vi "MaqEst.vi"() -> ()   [LabVIEW 2020]
uses:
  idle.ctl
panel:
  out "Dispensar":bool
  out "Enum 2":T1
  out "Dar Cambio":bool
  in  "Selected":bool
  in  "Coin Inserted":bool
  in  "Enough Coins":bool
  in  "Cancel":bool
  in  "Reject coins":bool
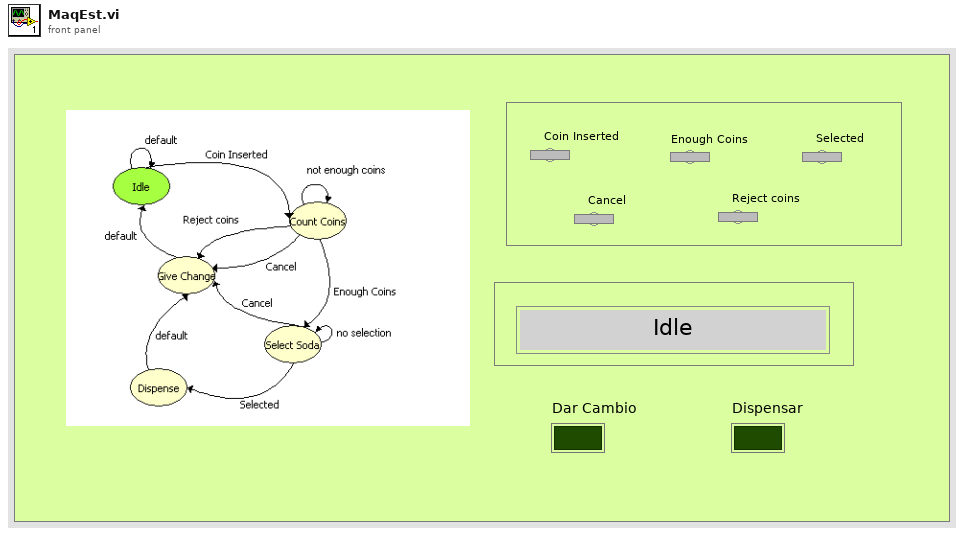
[diagram p1: front panel]
types:
  T1 = typedef "idle.ctl" = enum16{"Idle", "Count Coins", "Give Change", "Select Soda", "Dispense"}
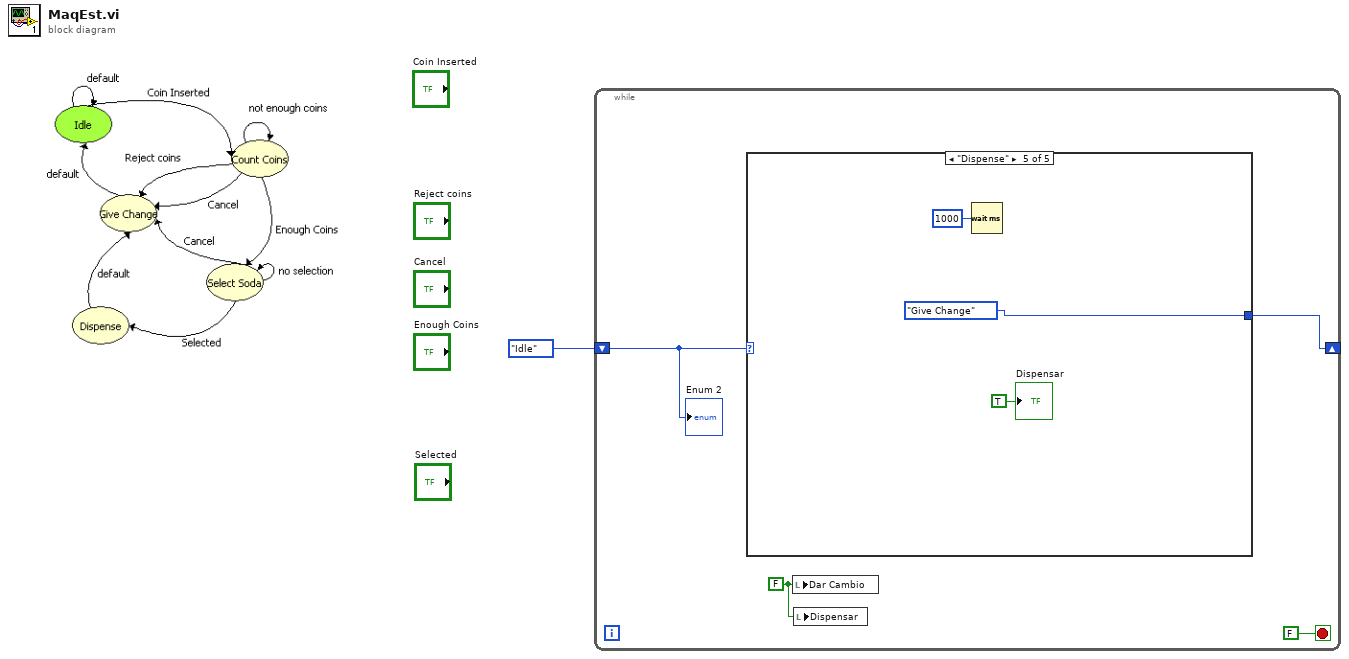
[diagram p0: block diagram]
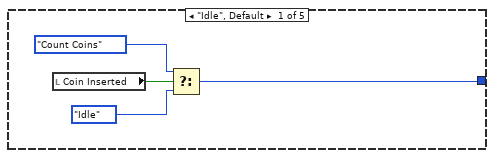
[diagram p2: hidden frame]
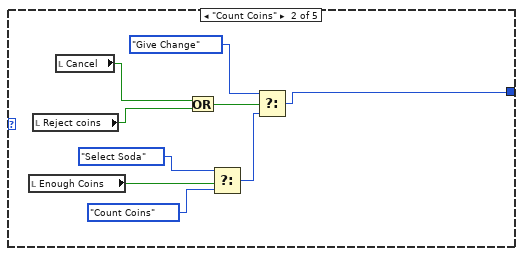
[diagram p3: hidden frame]
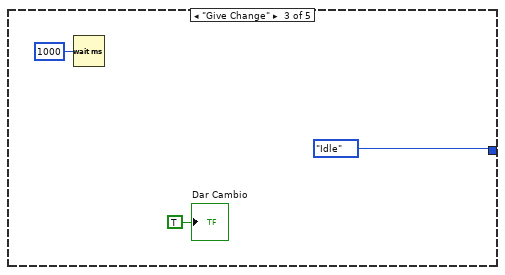
[diagram p4: hidden frame]
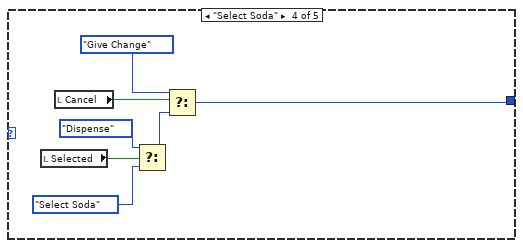
[diagram p5: hidden frame]
diagram:
  n1 = while {
    shift-right: [w4] -> _
    shift-left: idle."Idle" -> [w2]
    stop <- FALSE stop-if-true
    w3 = FALSE ("Dar Cambio")
    n2 = case shown="\"Dispense\"" w2 {
      tunnel: [w6 w10 idle."Idle" w22 idle."Give Change"] -> w4
      frame "Idle", Default {
        n3 = local read "Coin Inserted"() -> (w9:bool)
        n4 = Select(t=idle."Count Coins", s=w9, f=idle."Idle") -> (s? t:f=w6:T1)
      }
      frame "Count Coins" {
        n5 = local read "Enough Coins"() -> (w14:bool)
        n6 = local read "Reject coins"() -> (w17:bool)
        n7 = local read "Cancel"() -> (w18:bool)
        n8 = Or(x=w18, y=w17) -> (x .or. y?=w16:bool)
        n9 = Select(t=idle."Select Soda", s=w14, f=idle."Count Coins") -> (s? t:f=w12:T1)
        n10 = Select(t=idle."Give Change", s=w16, f=w12) -> (s? t:f=w10:T1)
      }
      frame "Give Change" {
        n11 = Wait (ms)(milliseconds to wait=u32 1000) -> ()  [unwired: 1 out]
        "Dar Cambio" <- TRUE ("Dar Cambio")
      }
      frame "Select Soda" {
        n12 = local read "Selected"() -> (w26:bool)
        n13 = local read "Cancel"() -> (w28:bool)
        n14 = Select(t=idle."Dispense", s=w26, f=idle."Select Soda") -> (s? t:f=w23:T1)
        n15 = Select(t=idle."Give Change", s=w28, f=w23) -> (s? t:f=w22:T1)
      }
      frame "Dispense" {
        n16 = Wait (ms)(milliseconds to wait=u32 1000) -> ()  [unwired: 1 out]
        "Dispensar" <- TRUE ("Dispensar")
      }
    }
    n17 = local write "Dar Cambio"(w3) -> ()
    n18 = local write "Dispensar"(w3) -> ()
    "Enum 2" <- w2
  }
